vi "To Log File.vi"(7 "new line":bool=TRUE, 8 "error in (no error)":errorcluster, 11 "string":string) -> (0 "error out":errorcluster)   [LabVIEW 2014, in "lvprj2html.lvlib"]
uses:
  lvprj2html.lvlib
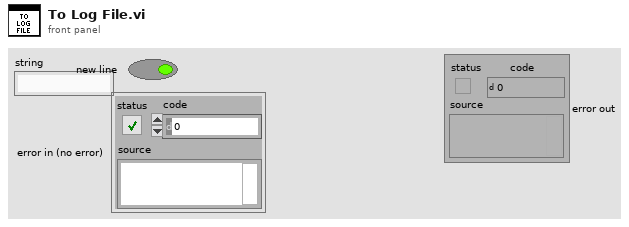
[diagram p1: front panel]
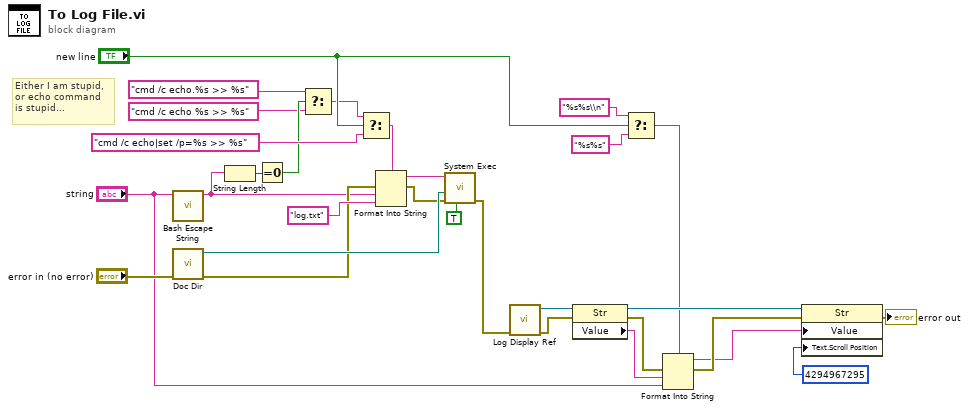
[diagram p0: block diagram]
diagram:
  # "Either I am stupid,\nor echo command\nis stupid..."
  n1 = call "Bash Escape String.vi"("string in"="string") -> ("string out"=w6:string)  [unwired: 10 in]
  n2 = call "Doc Dir.vi"("error in (no error)"="error in (no error)") -> ("error out"=w7:errorcluster, "appended path"=w28:path)  [unwired: 9 in]
  n3 = String Length(string=w6) -> (length=w5:i32)
  n4 = Equal To 0?(x=w5) -> (x = 0?=w3:bool)
  n5 = Select(t="cmd /c echo.%s >> %s" ("format string"), s=w3, f="cmd /c echo %s >> %s" ("format string")) -> (s? t:f=w4:string)
  n6 = Select(t=w4, s="new line", f="cmd /c echo|set /p=%s >> %s" ("format string")) -> (s? t:f=w13:string)
  n7 = Format Into String(format string=w13, error in=w7, w6, "log.txt" ("input 2")) -> (resulting string=w29:string, error out=w26:errorcluster)  [unwired: 1 in]
  n8 = call <vilib>:"System Exec.vi"("run minimized? (F)"=TRUE, "error in (no error)"=w26, "working directory"=w28, "command line"=w29) -> ("error out"=w25:errorcluster)  [unwired: 4 in, 3 out]
  n9 = call "Log Display Ref.vi"("error in"=w25) -> ("error out"=w18:errorcluster, "log display ref out"=w24:refnum<vi>)  [unwired: 9 in]
  n10 = property on="Property Node" class="Str"(reference=w24, error in=w18) -> (reference out=w23:refnum<vi>, error out=w21:errorcluster, "Value"=w20:string)
  n11 = Select(t="%s%s\\n" ("format string"), s="new line", f="%s%s" ("format string")) -> (s? t:f=w10:string)
  n12 = Format Into String(format string=w10, error in=w21, w20, "string") -> (resulting string=w19:string, error out=w22:errorcluster)  [unwired: 1 in]
  n13 = property on="Property Node" class="Str"(reference=w23, error in=w22, "Value"=w19, "Text.Scroll Position"=u32 4294967295) -> (error out=→"error out":errorcluster)  [unwired: 1 out]
